vi "createCommand.vi"(8 "error in (no error)":errorcluster, 10 "Command":T1, 11 "CommandFactory in":refnum<class "CommandFactory.lvclass">) -> (0 "error out":errorcluster, 2 "command":refnum<class "Command.lvclass">, 3 "CommandFactory out":refnum<class "CommandFactory.lvclass">)   [LabVIEW 2012, in "CommandFactory.lvclass"]
uses:
  CommandFactory.lvclass
  Command/Command.lvclass
  Typedefs/CommandSelector.ctl
  Commands/ClearError/ClearError.lvclass
  Commands/Exit/Exit.lvclass
  Commands/StandBy/StandBy.lvclass
  Commands/Start/Start.lvclass
  Commands/SwitchToOnDemandMode/SwitchToOnDemandMode.lvclass
  Commands/SwitchToStreamMode/SwitchToStreamMode.lvclass
  Commands/Update/Update.lvclass
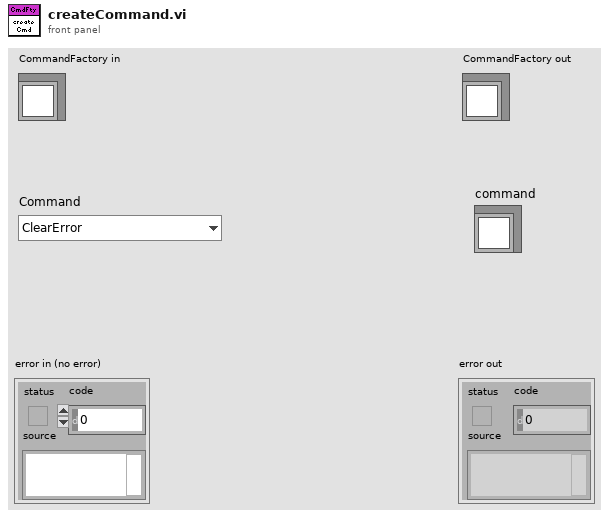
[diagram p1: front panel]
types:
  T1 = typedef "CommandSelector.ctl" = enum16{"ClearError", "Exit", "StandBy", "Start", "SwitchToOnDemandMode", "SwitchToStreamMode", "Update"}
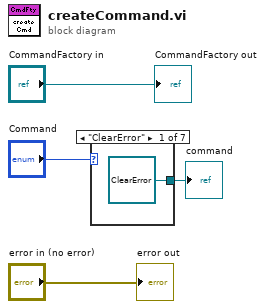
[diagram p0: block diagram]
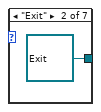
[diagram p2: hidden frame]
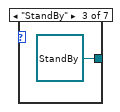
[diagram p3: hidden frame]
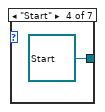
[diagram p4: hidden frame]
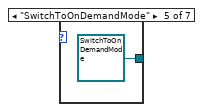
[diagram p5: hidden frame]
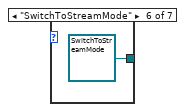
[diagram p6: hidden frame]
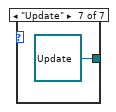
[diagram p7: hidden frame]
diagram:
  n1 = case shown="\"ClearError\"" "Command" {
    tunnel: [refnum<class "ClearError.lvclass"> refnum ("ClearError.lvclass") refnum<class "Exit.lvclass"> refnum ("Exit.lvclass") refnum<class "StandBy.lvclass"> refnum ("StandBy.lvclass") refnum<class "Start.lvclass"> refnum ("Start.lvclass") refnum<class "SwitchToOnDemandMode.lvclass"> refnum ("SwitchToOnDemandMode.lvclass") refnum<class "SwitchToStreamMode.lvclass"> refnum ("SwitchToStreamMode.lvclass") refnum<class "Update.lvclass"> refnum ("Update.lvclass")] -> w2
    frame "ClearError" {
    }
    frame "Exit" {
    }
    frame "StandBy" {
    }
    frame "Start" {
    }
    frame "SwitchToOnDemandMode" {
    }
    frame "SwitchToStreamMode" {
    }
    frame "Update" {
    }
  }
  "command" <- w2
  "error out" <- "error in (no error)"
  "CommandFactory out" <- "CommandFactory in"
